vi "VisBx Anzeige PNS.vi"() -> ()   [LabVIEW 2015, in "Anlagenuebersicht.lvlib"]
uses:
  Seiten/Anlagenuebersicht/VisBx Anzeige/Anlagenuebersicht.lvlib
  Seiten/Anlagenuebersicht/VisBx Anzeige/VisBx Anzeige.lvlib
  <vilib>/Utility/miscctls.llb/LVPointTypeDef.ctl
  Seiten/Anlagenuebersicht/VisBx Anzeige/TDMS laden/TDMS laden.lvlib
  Allgemein/allgemeine Sub-VIs.lvlib
  cRIO/PC/Kommunikation mit cRIO.lvlib
  PNS/PNS.lvlib
  PNS/Aktionen FGV Istwerte.ctl
  PNS/PNS Ausgabefelder einfaerben Aktionen.ctl
  PNS/Aktionen FGV Grenzwerte.ctl
  Seiten/System Einstellungen/System Einstellungen.lvlib
  Seiten/System Einstellungen/Aktioen FGV System.ctl
  Stoerungen/Stoerungen.lvlib
  <vilib>/picture/picture.llb/Draw True-Color Pixmap.vi
  Funktionstasten/Funktionstasten.lvlib
  Funktionstasten/FGV Erweiterte Bedienung Aktion.ctl
  Visualisierungs Elemente/Zahlen-Ausgabefeld.ctl
panel:
  in  "Züruck zu Anlagenübersicht":bool
  out "Filter VFS 4":T1 caption="Filter:" format="%.1f"
  out "Filter VFS 3":T1 caption="Filter:" format="%.1f"
  out "Filter VFS 2":T1 caption="Filter:" format="%.1f"
  out "Filter VFS 1":T1 caption="Filter:" format="%.1f"
  out "HL1 VFS4":T1 caption="HL 1:" format="%.1f"
  out "HL1 VFS3":T1 caption="HL 1:" format="%.1f"
  out "HL 1 VFS2":T1 caption="HL 1:" format="%.1f"
  out "TRE HL 3":T1 caption="HL 3:" format="%.1f"
  out "TRE HL 2":T1 caption="HL 2:" format="%.1f"
  out "TRE HL 1":T1 caption="HL 1:" format="%.1f"
  out "TRE HL 6":T1 caption="HL 6:" format="%.1f"
  out "TRE HL 5":T1 caption="HL 5:" format="%.1f"
  out "HL1 VFS 1":T1 caption="HL 1:" format="%.1f"
  out "TRE HL 4":T1 caption="HL 4:" format="%.1f"
  out "Aktive Störungen":string[](array[string]) caption="Errors"
  out "Betriebsstunden Anlage:":T1 caption="Operating hours (unit):" format="%.1f"
  out "Betriebsstunden Pumpe:":T1 caption="Operating hours (measure):" format="%.1f"
  in  "Fehler":string="Die Umgebungsvariable besitzt\nnicht den selben Datentyp wie\ndie TDMS-Datei."
  out "Bild":picture
  # "Process Chart"
  # "GN2...Nitrogen gaseous\nCA.....Compressed air\nCG.....Cal. Gas\nAA.....Ambient air\nPA.....Purge air FT-IR\n\nPR....Pressure regulator\nPS....Pressure switch\nFS....Flow controller\nLS....Levelsensor\nFM...Flow Sensor"
  # "VFS 1.1"
  # "-11Y2"
  # "°C"
  # "-11Y5"
  # "SP1"
  # "VFS 1.1"
  # "-11Y3"
  # "-12Y1"
  # "°C"
  # "Panel"
  # "VFS 1.2"
  # "-11Y2"
  # "°C"
  # "-11Y5"
  # "SP2"
  # "VFS 1.2"
  # "-11Y3"
  # "-12Y1"
  # "Panel"
  # "1"
  # "VFS 1.3"
  # "-11Y2"
  # "°C"
  # "-11Y5"
  # "SP3"
  # "VFS 1.3"
  # "°C"
  # "-11Y3"
  # "-12Y1"
  # "VFS 1.4"
  # "h"
  # "-11Y2"
  # "°C"
  # "-11Y5"
  # "h"
  # "SP4"
  # "VFS 1.4"
  # "-11Y3"
  # "-12Y1"
  # "°C"
  # "°C"
  # "°C"
  # "°C"
  # "°C"
  # "°C"
  # "°C"
  # "CG"
  # "PNS"
  # "CA"
  # "PNS"
  # "CG"
  # "PNS"
  # "CA"
  # "PNS"
  # "CG"
  # "PNS"
  # "CA"
  # "PNS"
  # "CG"
  # "PNS"
  # "CA"
  # "PNS"
  # "°C"
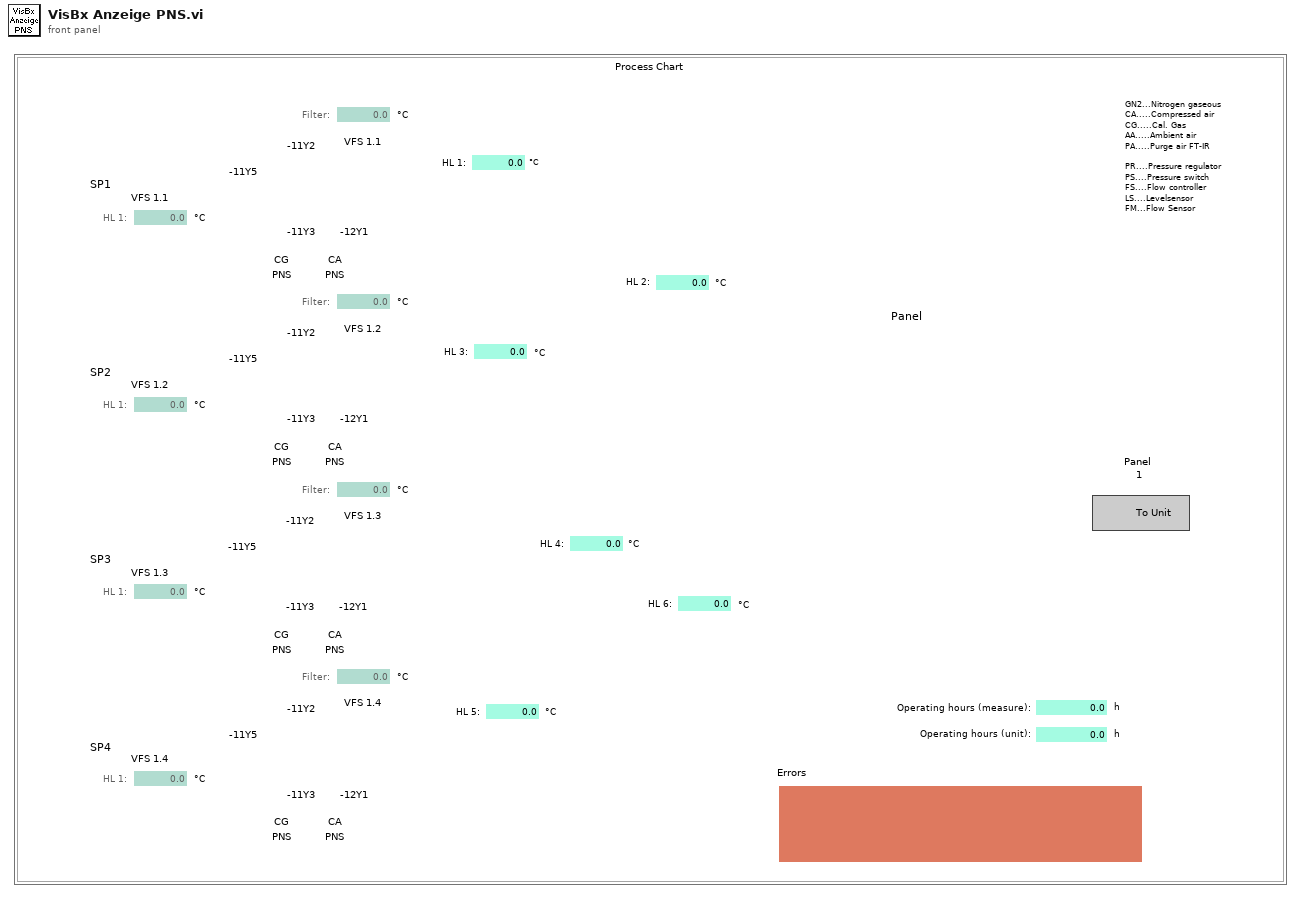
[diagram p1: front panel]
types:
  T1 = typedef "Zahlen-Ausgabefeld.ctl" = sgl
  T2 = typedef "Funktionstasten.lvlib/FGV Erweiterte Bedienung Aktion.ctl" = enum16{"Lesen", "Initialisieren", "N2 zu PNS", "Chart wechsel"}
  T3 = typedef "PNS.lvlib/Aktionen FGV Grenzwerte.ctl" = enum16{"lesen", "Grenzw. schreiben", "Anweisungscode"}
  T4 = typedef "System Einstellungen.lvlib/Aktioen FGV System.ctl" = enum16{"lesen", "laden", "speichern", "Optionen schreiben", "Zeitstempel", "Reset BMP", "Reset SQP", "Wartung"}
  T5 = typedef "PNS.lvlib/PNS Ausgabefelder einfaerben Aktionen.ctl" = enum16{"lesen", "prüfen", "initialisieren"}
  T6 = typedef "LVPointTypeDef.ctl" = cluster{"Horizontal":i16, "Vertical":i16}
  T7 = enum8{"Enabled", "Disabled", "Disabled and Grayed Out"}
  T8 = typedef "PNS.lvlib/Anlagengrenzwerte PNS.ctl" = cluster{"Filter:":T9, "Ventilplatte:":T9, "Heizleitung 1:":T9, "Heizleitung 2:":T9, "Heizleitung 3:":T9, "Heizleitung 4:":T9, "Heizleitung 5:":T9, "Heizleitung 6:":T9}
  T9 = typedef "PNS.lvlib/Anlagengrenzwerte-Parameter Anzeige.ctl" = cluster{"Sollwert":T10, "Warn-Min":T10, "Warn-Max":T10, "Abschalt-Min":T10, "Abschalt-Max":T10, "Regler":u16, "AnlagenParameter":string}
  T10 = typedef "Zahlen-Eingabefeld.ctl" = sgl
  T11 = typedef "System Einstellungen.lvlib/Optionen.ctl" = cluster{"Störmeldep.":bool, "Betriebszustände":bool, "LN2 Befüllung":bool, "Klimaanlage ?":bool, "AK in ppm":bool, "log Cal-Gas":bool, "log 0-Gas":bool, "log CG zu PNS":bool, "Reserve":bool, "Reserve1":bool, "PNS?":bool, "Container":bool, "Mit N2 spülen":bool, "Span Gas Auswahl":T12, "VFS 1":bool, "VFS 2":bool, "VFS 3":bool, "VFS 4":bool, "TRE08":bool}
  T12 = typedef "Funktionstasten.lvlib/Spaneingang.ctl" = u16
  T13 = typedef "VisParam-Typdef.lvlib/VisSchritt.ctl" = cluster{"Schritt-Typ":T14, "Schritt-Daten":variant}
  T14 = typedef "VisParam-Typdef.lvlib/VisSchritt-Typ.ctl" = enum16{"leer", "Punkt", "Linie", "Linienzug", "Fixtext", "Textrechteck", "Ziffernanzeige", "Rechteck", "Rechteck rund", "Ellipse", "Bogen", "Kreis", "Pixmap"}
  T15 = typedef "Anlagenuebersicht.lvlib/VisBx Anzeige.lvlib/TDMS laden.lvlib/TDMS-Eigenschaften.ctl" = cluster{"Größe":T16, "URL":string, "Raster":i16, "Hintergrund":u32}
  T16 = typedef "LVBoundsTypeDef.ctl" = cluster{"Width":u32, "Height":u32}
  T17 = typedef "PNS.lvlib/Aktionen FGV Istwerte.ctl" = enum16{"lesen", "Regler", "Alarme", "UsrVal", "initialisieren"}
  T18 = typedef "PNS.lvlib/Komm Modbus.lvlib/Modbus TypDef.lvlib/Regler.ctl" = cluster{"Istwert":i16, "Sollwert":i16, "Alarm MIN":i16, "Alarm MAX":i16, "Regler sperren":i16, "Analog Ausgang":i16}
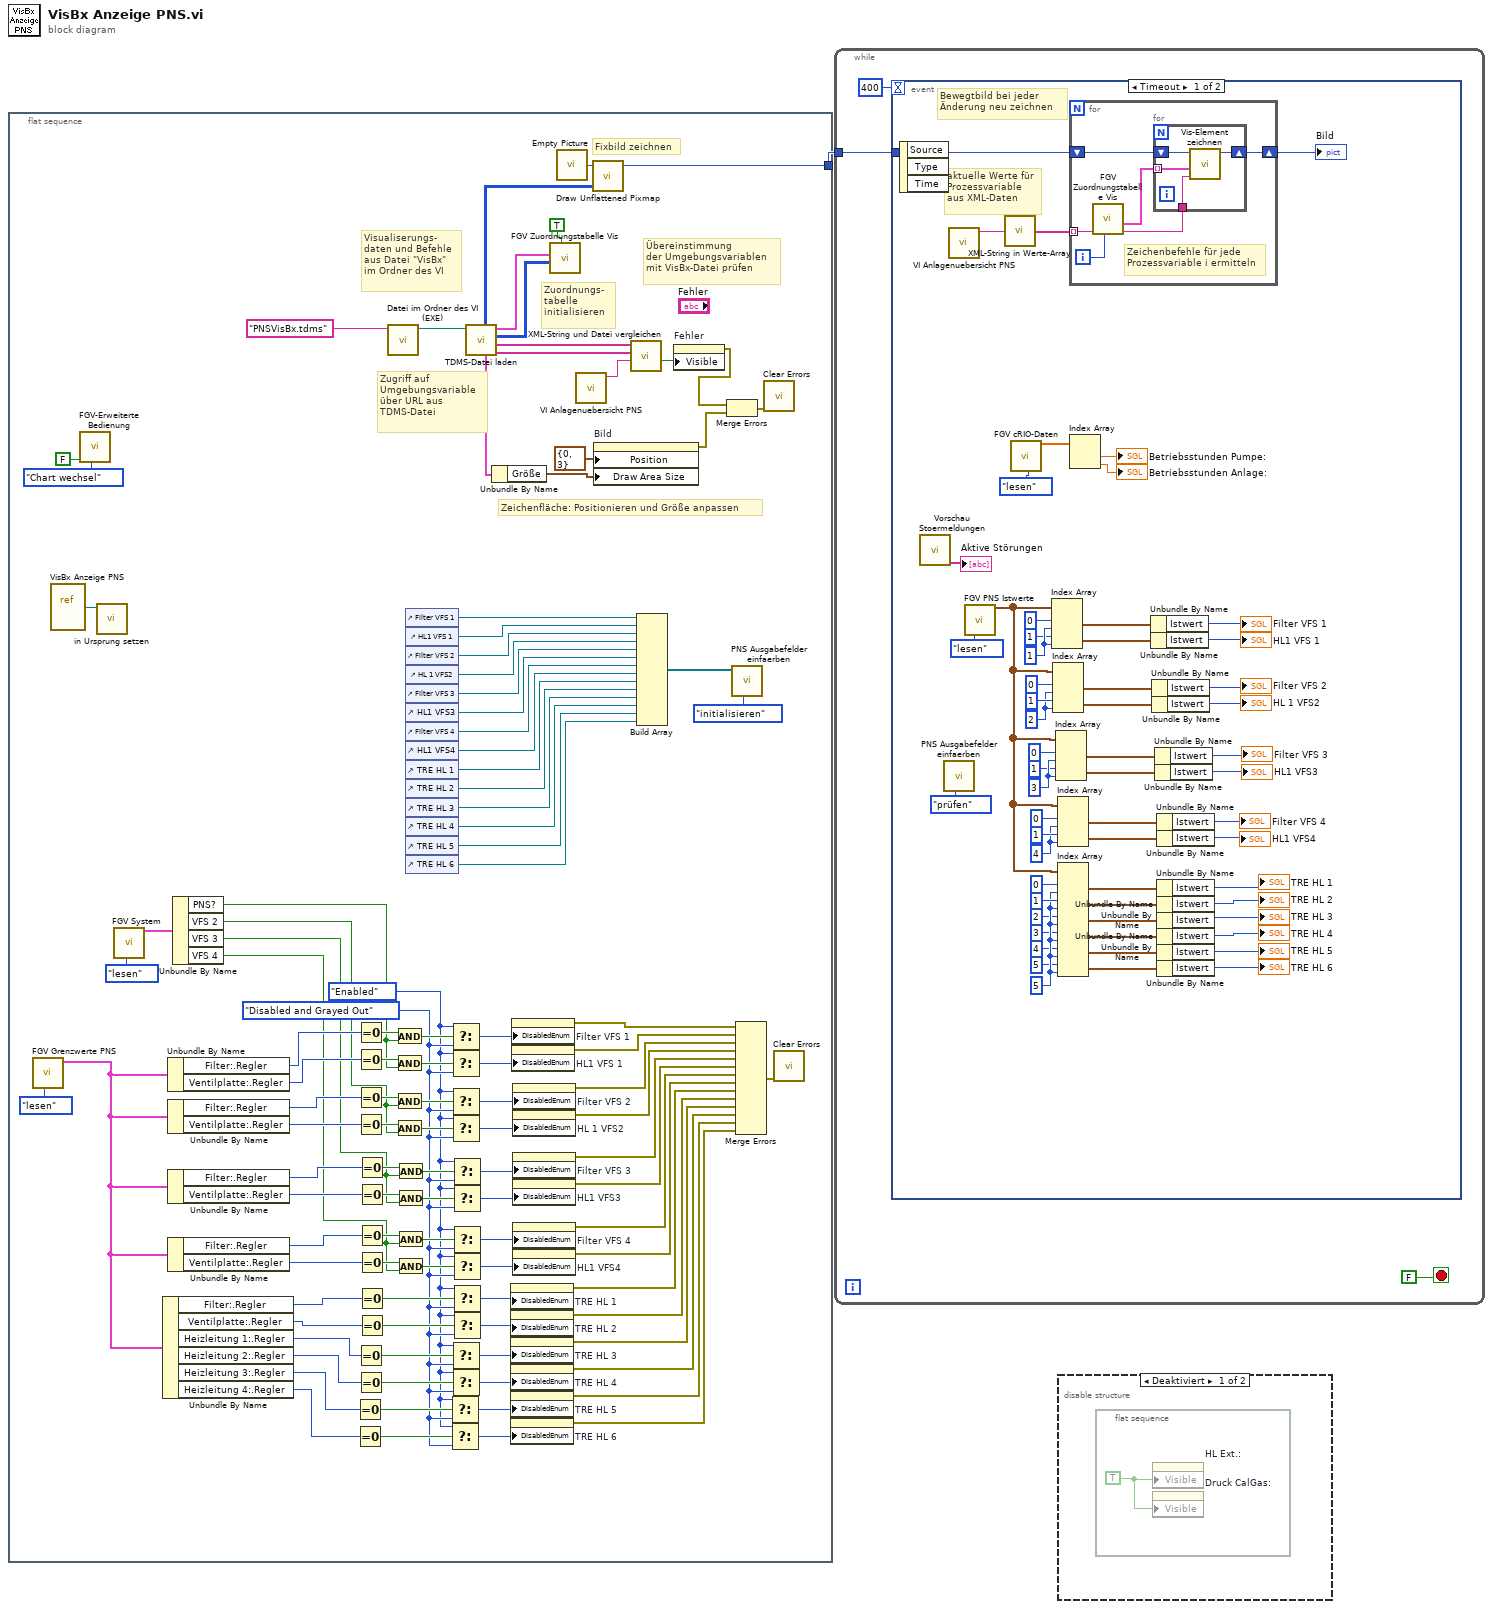
[diagram p0: block diagram]
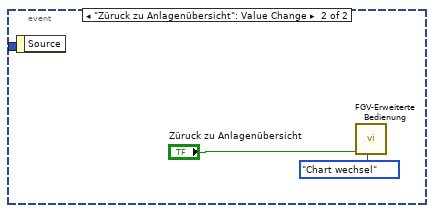
[diagram p3: hidden frame]
diagram:
  n1 = flat-sequence {
    tunnel: [w99] -> w1
    frame #0 {
      w42 = T7."Enabled" ("t")
      w43 = T7."Disabled and Grayed Out" ("Deaktiviert")
      # "Übereinstimmung\nder Umgebungsvariablen\nmit VisBx-Datei prüfen"
      # "Zugriff auf\nUmgebungsvariable\nüber URL aus\nTDMS-Datei"
      # "Visualiserungs-\ndaten und Befehle\naus Datei \"VisBx\"\nim Ordner des VI"
      # "Zuordnungs-\ntabelle\ninitialisieren"
      # "Zeichenfläche: Positionieren und Größe anpassen"
      # "Fixbild zeichnen"
      n2 = call "FGV Grenzwerte PNS.vi"("Aktionen FGV Grenzwerte"=Aktionen_FGV_Grenzwerte."lesen") -> ("Grenzwerte PNS"=w2:T8)  [unwired: 9 in, 1 out]
      n3 = vi-ref "VisBx Anzeige PNS.vi"() -> (w113:refnum<vi>)
      n4 = call "FGV-Erweiterte Bedienung.vi"("Aktion"=FGV_Erweiterte_Bedienung_Aktion."Chart wechsel", "Chart wechsel"=FALSE) -> ()  [unwired: 8 in, 2 out]
      n5 = call "in Ursprung setzen.vi"("VI Referenz"=w113) -> ()  [unwired: 11 in]
      n6 = call "FGV System.vi"("Aktionen"=Aktioen_FGV_System."lesen") -> ("Optionen"=w67:T11)  [unwired: 13 in, 5 out]
      n7 = Unbundle By Name(w2) -> ("Filter:.Regler"=w41:u16, "Ventilplatte:.Regler"=w40:u16, "Heizleitung 1:.Regler"=w39:u16, "Heizleitung 2:.Regler"=w38:u16, "Heizleitung 3:.Regler"=w37:u16, "Heizleitung 4:.Regler"=w36:u16)
      n8 = Unbundle By Name(w2) -> ("Filter:.Regler"=w73:u16, "Ventilplatte:.Regler"=w65:u16)
      n9 = Unbundle By Name(w2) -> ("Filter:.Regler"=w64:u16, "Ventilplatte:.Regler"=w63:u16)
      n10 = Unbundle By Name(w2) -> ("Filter:.Regler"=w58:u16, "Ventilplatte:.Regler"=w57:u16)
      n11 = Unbundle By Name(w2) -> ("Filter:.Regler"=w52:u16, "Ventilplatte:.Regler"=w51:u16)
      n12 = Unbundle By Name(w67) -> ("PNS?"=w44:bool, "VFS 2"=w19:bool, "VFS 3"=w18:bool, "VFS 4"=w17:bool)
      n13 = Equal To 0?(x=w37) -> (x = 0?=w45:bool)
      n14 = Equal To 0?(x=w36) -> (x = 0?=w46:bool)
      n15 = Equal To 0?(x=w73) -> (x = 0?=w72:bool)
      n16 = Equal To 0?(x=w65) -> (x = 0?=w71:bool)
      n17 = Equal To 0?(x=w64) -> (x = 0?=w70:bool)
      n18 = Equal To 0?(x=w63) -> (x = 0?=w69:bool)
      n19 = Equal To 0?(x=w39) -> (x = 0?=w48:bool)
      n20 = Equal To 0?(x=w38) -> (x = 0?=w47:bool)
      n21 = Equal To 0?(x=w58) -> (x = 0?=w61:bool)
      n22 = Equal To 0?(x=w57) -> (x = 0?=w62:bool)
      n23 = Equal To 0?(x=w52) -> (x = 0?=w54:bool)
      n24 = Equal To 0?(x=w51) -> (x = 0?=w53:bool)
      n25 = Equal To 0?(x=w41) -> (x = 0?=w49:bool)
      n26 = Equal To 0?(x=w40) -> (x = 0?=w50:bool)
      n27 = call "Datei im Ordner des VI (EXE).vi"("Dateiname"="PNSVisBx.tdms") -> ("Dateipfad im Ordner des Haupt-VIs"=w112:path)  [unwired: 8 in, 2 out]
      n28 = And(x=w72, y=w44) -> (x .and. y?=w94:bool)
      n29 = And(x=w71, y=w44) -> (x .and. y?=w93:bool)
      n30 = And(x=w70, y=w19) -> (x .and. y?=w92:bool)
      n31 = And(x=w69, y=w19) -> (x .and. y?=w91:bool)
      n32 = And(x=w61, y=w18) -> (x .and. y?=w59:bool)
      n33 = And(x=w62, y=w18) -> (x .and. y?=w60:bool)
      n34 = And(x=w54, y=w17) -> (x .and. y?=w56:bool)
      n35 = And(x=w53, y=w17) -> (x .and. y?=w55:bool)
      n36 = control-ref of="Filter VFS 1"() -> (w87:refnum<vi>)
      n37 = control-ref of="HL1 VFS 1"() -> (w86:refnum<vi>)
      n38 = control-ref of="Filter VFS 2"() -> (w85:refnum<vi>)
      n39 = control-ref of="HL 1 VFS2"() -> (w84:refnum<vi>)
      n40 = control-ref of="Filter VFS 3"() -> (w83:refnum<vi>)
      n41 = control-ref of="HL1 VFS3"() -> (w82:refnum<vi>)
      n42 = control-ref of="Filter VFS 4"() -> (w81:refnum<vi>)
      n43 = control-ref of="HL1 VFS4"() -> (w80:refnum<vi>)
      n44 = control-ref of="TRE HL 1"() -> (w79:refnum<vi>)
      n45 = control-ref of="TRE HL 2"() -> (w78:refnum<vi>)
      n46 = control-ref of="TRE HL 3"() -> (w77:refnum<vi>)
      n47 = control-ref of="TRE HL 4"() -> (w76:refnum<vi>)
      n48 = control-ref of="TRE HL 5"() -> (w75:refnum<vi>)
      n49 = control-ref of="TRE HL 6"() -> (w74:refnum<vi>)
      n50 = Select(t=w42, s=w45, f=w43) -> (s? t:f=w12:T7)
      n51 = Select(t=w42, s=w46, f=w43) -> (s? t:f=w11:T7)
      n52 = Select(t=w42, s=w94, f=w43) -> (s? t:f=w35:T7)
      n53 = Select(t=w42, s=w93, f=w43) -> (s? t:f=w33:T7)
      n54 = Select(t=w42, s=w92, f=w43) -> (s? t:f=w31:T7)
      n55 = Select(t=w42, s=w91, f=w43) -> (s? t:f=w30:T7)
      n56 = Select(t=w42, s=w48, f=w43) -> (s? t:f=w14:T7)
      n57 = Select(t=w42, s=w47, f=w43) -> (s? t:f=w13:T7)
      n58 = Select(t=w42, s=w59, f=w43) -> (s? t:f=w27:T7)
      n59 = Select(t=w42, s=w60, f=w43) -> (s? t:f=w26:T7)
      n60 = Select(t=w42, s=w56, f=w43) -> (s? t:f=w23:T7)
      n61 = Select(t=w42, s=w55, f=w43) -> (s? t:f=w22:T7)
      n62 = Select(t=w42, s=w49, f=w43) -> (s? t:f=w16:T7)
      n63 = Select(t=w42, s=w50, f=w43) -> (s? t:f=w15:T7)
      n64 = call "TDMS-Datei laden.vi"("Dateipfad"=w112) -> ("Datentypen"=w108:string[], "Namen"=w104:string[], "Zuordnungstabelle"=w102:i16[][], "Programm"=w103:T13[], "Eigenschaften"=w105:T15, "Fixbild (Pixmap)"=w106:u32[][])  [unwired: 5 out]
      n65 = Unbundle By Name(w105) -> ("Größe"=w111:T16)
      n66 = property on="TRE HL 1" class="DigWert (strikt)"("DisabledEnum"=w16) -> (error out=w10:errorcluster)  [unwired: 2 in, 1 out]
      n67 = property on="TRE HL 2" class="DigWert (strikt)"("DisabledEnum"=w15) -> (error out=w9:errorcluster)  [unwired: 2 in, 1 out]
      n68 = property on="TRE HL 3" class="DigWert (strikt)"("DisabledEnum"=w14) -> (error out=w8:errorcluster)  [unwired: 2 in, 1 out]
      n69 = property on="TRE HL 4" class="DigWert (strikt)"("DisabledEnum"=w13) -> (error out=w7:errorcluster)  [unwired: 2 in, 1 out]
      n70 = property on="TRE HL 5" class="DigWert (strikt)"("DisabledEnum"=w12) -> (error out=w6:errorcluster)  [unwired: 2 in, 1 out]
      n71 = property on="TRE HL 6" class="DigWert (strikt)"("DisabledEnum"=w11) -> (error out=w5:errorcluster)  [unwired: 2 in, 1 out]
      n72 = property on="Filter VFS 1" class="DigWert (strikt)"("DisabledEnum"=w35) -> (error out=w34:errorcluster)  [unwired: 2 in, 1 out]
      n73 = property on="HL1 VFS 1" class="DigWert (strikt)"("DisabledEnum"=w33) -> (error out=w32:errorcluster)  [unwired: 2 in, 1 out]
      n74 = property on="Filter VFS 2" class="DigWert (strikt)"("DisabledEnum"=w31) -> (error out=w29:errorcluster)  [unwired: 2 in, 1 out]
      n75 = property on="HL 1 VFS2" class="DigWert (strikt)"("DisabledEnum"=w30) -> (error out=w28:errorcluster)  [unwired: 2 in, 1 out]
      n76 = property on="Filter VFS 3" class="DigWert (strikt)"("DisabledEnum"=w27) -> (error out=w25:errorcluster)  [unwired: 2 in, 1 out]
      n77 = property on="HL1 VFS3" class="DigWert (strikt)"("DisabledEnum"=w26) -> (error out=w24:errorcluster)  [unwired: 2 in, 1 out]
      n78 = property on="Filter VFS 4" class="DigWert (strikt)"("DisabledEnum"=w23) -> (error out=w21:errorcluster)  [unwired: 2 in, 1 out]
      n79 = property on="HL1 VFS4" class="DigWert (strikt)"("DisabledEnum"=w22) -> (error out=w20:errorcluster)  [unwired: 2 in, 1 out]
      n80 = call "FGV Zuordnungstabelle Vis.vi"("Initialisieren"=TRUE, "Zuordnungtabelle (init)"=w102, "Programm (init)"=w103) -> ()  [unwired: 3 in, 6 out]
      n81 = call "Empty Picture"() -> ("empty picture"=w107:picture)
      n82 = call "VI Anlagenuebersicht PNS.vi"() -> ("XML-String"=w109:string)  [unwired: 11 in]
      n83 = call-poly <vilib>:"Draw Unflattened Pixmap.vi"("picture"=w107, "data (RGB format)"=w106) -> ("new picture"=w99:picture)  [unwired: 7 in]
      n84 = property on="Bild" class="Bild"("Position"=T6 {"Horizontal"=0, "Vertical"=3} ("Ursprung"), "Draw Area Size"=w111) -> (error out=w95:errorcluster)  [unwired: 2 in, 1 out]
      n85 = call "XML-String und Datei vergleichen.vi"("XML-String"=w109, "Datentypen aus Datei"=w108, "Namen aus Datei"=w104) -> ("nicht gleich"=w101:bool)  [unwired: 8 out]
      n86 = Build Array(w87, w86, w85, w84, w83, w82, w81, w80, w79, w78, w77, w76, w75, w74) -> (w88:refnum<vi>[])
      n87 = property on="Fehler" class="Str"("Visible"=w101) -> (error out=w96:errorcluster)  [unwired: 2 in, 1 out]
      n88 = Merge Errors(w96, w95) -> (w97:errorcluster)
      n89 = call "PNS Ausgabefelder einfaerben.vi"("Aktionen"=PNS_Ausgabefelder_einfaerben_Aktionen."initialisieren", "Angehängtes Array"=w88) -> ()  [unwired: 10 in]
      n90 = Merge Errors(w34, w32, w29, w28, w25, w24, w21, w20, w10, w9, w8, w7, w6, w5) -> (w98:errorcluster)
      n91 = call <vilib>:"Clear Errors.vi"("error in (no error)"=w97) -> ()  [unwired: 5 in, 2 out]
      n92 = call <vilib>:"Clear Errors.vi"("error in (no error)"=w98) -> ()  [unwired: 5 in, 2 out]
    }
  }
  n93 = while {
    tunnel: w1 -> [w116]
    stop <- FALSE stop-if-true
    n94 = event shown="[0] Timeout" {
      selector: _ -> [_ _]
      dyn-events: _ -> [_ _]
      timeout: 400 -> [_ _]
      tunnel: w116 -> [w175 _]
      event Timeout {
        w140 = 5 ("Deaktivierter Index (Spalte)")
        w148 = 4 ("Deaktivierter Index (Spalte)")
        w151 = 3 ("Deaktivierter Index (Spalte)")
        w158 = 2 ("Deaktivierter Index (Spalte)")
        w161 = 1 ("Deaktivierter Index (Spalte)")
        # "aktuelle Werte für\nProzessvariable\naus XML-Daten"
        # "Bewegtbild bei jeder\nÄnderung neu zeichnen"
        n95 = event-data() -> ()  [unwired: 1 in, 3 out]
        n96 = call "Vorschau Stoermeldungen.vi"() -> ("Vorschau Störungen"=→"Aktive Störungen":string[])  [unwired: 10 in, 1 out]
        n97 = call "PNS Ausgabefelder einfaerben.vi"("Aktionen"=PNS_Ausgabefelder_einfaerben_Aktionen."prüfen") -> ()  [unwired: 11 in]
        n98 = call "VI Anlagenuebersicht PNS.vi"() -> ("XML-String"=w172:string)  [unwired: 11 in]
        n99 = call "FGV PNS Istwerte.vi"("Aktionen"=Aktionen_FGV_Istwerte."lesen") -> ("Regler"=w131:T18[])  [unwired: 12 in, 2 out]
        n100 = call "XML-String in Werte-Array.vi"("XML-String"=w172) -> ("Werte"=w173:string[])
        n101 = call "FGV cRIO-Daten.vi"("Aktion"=enum16{"lesen", "schreiben"}."lesen") -> ("Betriebsstunden"=w168:sgl[])  [unwired: 9 in, 9 out]
        n102 = Index Array(array=w131, index (row) #1=0 ("Deaktivierter Index (Zeile)"), index (col) #1=w161, index (row) #2=1 ("Deaktivierter Index (Zeile)"), index (col) #2=w161) -> (element #1=w164:T18, element #2=w163:T18)
        n103 = Index Array(array=w131, index (row) #1=0 ("Deaktivierter Index (Zeile)"), index (col) #1=w158, index (row) #2=1 ("Deaktivierter Index (Zeile)"), index (col) #2=w158) -> (element #1=w155:T18, element #2=w156:T18)
        n104 = Index Array(array=w131, index (row) #1=0 ("Deaktivierter Index (Zeile)"), index (col) #1=w151, index (row) #2=1 ("Deaktivierter Index (Zeile)"), index (col) #2=w151) -> (element #1=w154:T18, element #2=w153:T18)
        n105 = Index Array(array=w131, index (row) #1=0 ("Deaktivierter Index (Zeile)"), index (col) #1=w148, index (row) #2=1 ("Deaktivierter Index (Zeile)"), index (col) #2=w148) -> (element #1=w145:T18, element #2=w146:T18)
        n106 = Index Array(array=w131, index (row) #1=0 ("Deaktivierter Index (Zeile)"), index (col) #1=w140, index (row) #2=1 ("Deaktivierter Index (Zeile)"), index (col) #2=w140, index (row) #3=2 ("Deaktivierter Index (Zeile)"), index (col) #3=w140, index (row) #4=3 ("Deaktivierter Index (Zeile)"), index (col) #4=w140, index (row) #5=4 ("Deaktivierter Index (Zeile)"), index (col) #5=w140, index (row) #6=5 ("Deaktivierter Index (Zeile)"), index (col) #6=w140) -> (element #1=w144:T18, element #2=w143:T18, element #3=w139:T18, element #4=w138:T18, element #5=w137:T18, element #6=w136:T18)
        n107 = for {
          shift-right: [w181] -> w171
          shift-left: w175 -> [w178]
          tunnel: w173 -> [w177] mode=indexing
          i -> [w176]
          # "Zeichenbefehle für jede\nProzessvariable i ermitteln"
          n108 = call "FGV Zuordnungstabelle Vis.vi"("Prozessvariable Nr. N"=w176, "Wert (N)"=w177) -> ("Wert für zeichnen"=w179:string, "Zeichenbefehle"=w180:T13[])  [unwired: 4 in, 4 out]
          n109 = for {
            tunnel: w179 -> [w182]
            tunnel: w180 -> [w183] mode=indexing
            shift-right: [w185] -> w181
            shift-left: w178 -> [w184]
            n110 = call "Vis-Element zeichnen.vi"("Wert-String"=w182, "Schritt"=w183, "Bild alt"=w184) -> ("Bild neu"=w185:picture)  [unwired: 4 in, 4 out]
          }
        }
        "Bild" <- w171
        n111 = Index Array(array=w168) -> (element #1=→"Betriebsstunden Pumpe:":sgl, element #2=→"Betriebsstunden Anlage:":sgl)  [unwired: 2 in]
        n112 = Unbundle By Name(w164) -> ("Istwert"=→"Filter VFS 1":i16)
        n113 = Unbundle By Name(w163) -> ("Istwert"=→"HL1 VFS 1":i16)
        n114 = Unbundle By Name(w155) -> ("Istwert"=→"Filter VFS 2":i16)
        n115 = Unbundle By Name(w156) -> ("Istwert"=→"HL 1 VFS2":i16)
        n116 = Unbundle By Name(w154) -> ("Istwert"=→"Filter VFS 3":i16)
        n117 = Unbundle By Name(w153) -> ("Istwert"=→"HL1 VFS3":i16)
        n118 = Unbundle By Name(w145) -> ("Istwert"=→"Filter VFS 4":i16)
        n119 = Unbundle By Name(w146) -> ("Istwert"=→"HL1 VFS4":i16)
        n120 = Unbundle By Name(w144) -> ("Istwert"=→"TRE HL 1":i16)
        n121 = Unbundle By Name(w143) -> ("Istwert"=→"TRE HL 2":i16)
        n122 = Unbundle By Name(w139) -> ("Istwert"=→"TRE HL 3":i16)
        n123 = Unbundle By Name(w138) -> ("Istwert"=→"TRE HL 4":i16)
        n124 = Unbundle By Name(w137) -> ("Istwert"=→"TRE HL 5":i16)
        n125 = Unbundle By Name(w136) -> ("Istwert"=→"TRE HL 6":i16)
      }
      event "Züruck zu Anlagenübersicht": Value Change {
        n126 = event-data() -> ()  [unwired: 1 in, 1 out]
        n127 = call "FGV-Erweiterte Bedienung.vi"("Aktion"=FGV_Erweiterte_Bedienung_Aktion."Chart wechsel", "Chart wechsel"="Züruck zu Anlagenübersicht") -> ()  [unwired: 8 in, 2 out]
      }
    }
  }
  n128 = disable-structure shown="Deaktiviert" {
    frame Disabled {
      n129 = flat-sequence {
        frame #0 {
          w188 = TRUE ("Sichtbar")
          n130 = property on="HL Ext.:" class="DigWert (strikt)"("Visible"=w188) -> ()  [unwired: 2 in, 2 out]
          n131 = property on="Druck CalGas:" class="DigWert (strikt)"("Visible"=w188) -> ()  [unwired: 2 in, 2 out]
        }
      }
    }
    frame Enabled {
    }
  }
